vi "Terminal-ModbusEthernet-ReadInputRegisters.vi"(5 "write operation timeout (ms)":i32=5000 caption="写操作超时（毫秒）", 7 "read operation timeout (ms)":i32=5000 caption="读操作超时（毫秒）", 8 "error in":errorcluster, 9 "number of input registers":u16 caption="输入寄存器数量", 10 "starting address":u16 caption="起始地址", 11 "unit ID":u8 caption="单元ID") -> (0 "error out":errorcluster, 3 "register values":u16[](array[numeric]) caption="寄存器值")   [LabVIEW 2014]
uses:
  <vilib>/Modbus/subvis/Modbus API/Modbus API.lvclass/Modbus API.ctl
  <vilib>/Modbus/subvis/Transmission Data Unit (ADU)/Transmission Data Unit/Transmission Data Unit.lvclass/Transmission Data Unit.ctl
  <vilib>/Modbus/master/Data Access/Unit ID/Set Unit ID Property.vi
  <vilib>/Modbus/subvis/Transmission Data Unit (ADU)/Transmission Data Unit/Data Access/Unit ID/Write Unit ID.vi
  <vilib>/Modbus/subvis/Modbus API/Read Transmission Data Unit.vi
  <vilib>/Modbus/subvis/Modbus API/Write Transmission Data Unit.vi
  Configuration-Global.vi
  <vilib>/Modbus/master/Create Master Instance (TCP).vi
  <vilib>/Modbus/subvis/Transmission Data Unit (ADU)/Transmission Data Unit/Transmission Data Unit.lvclass
  <vilib>/Modbus/master/Modbus Master.lvclass
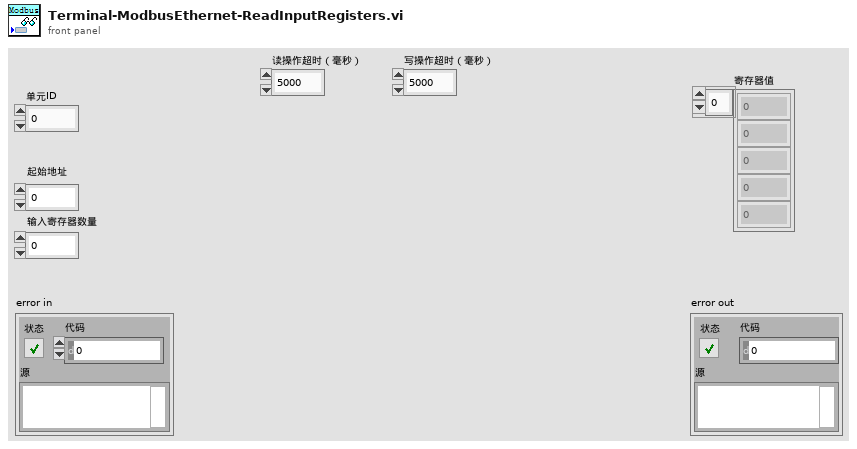
[diagram p1: front panel]
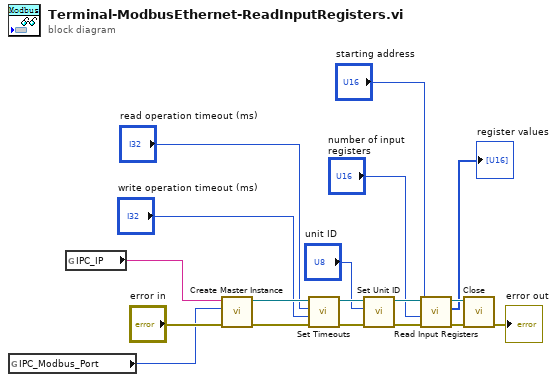
[diagram p0: block diagram]
diagram:
  n1 = global read "Configuration-Global.vi" "IPC_Modbus_Port"() -> (w4:i32)
  n2 = global read "Configuration-Global.vi" "IPC_IP"() -> (w5:string)
  n3 = call-poly <vilib>:"Create Master Instance.vi"("error in (no error)"="error in", "port (502)"=w4, "address"=w5) -> ("error out"=w16:errorcluster, "TCP master instance"=w15:refnum<class "Modbus Master.lvclass">)  [unwired: 7 in]
  n4 = call <vilib>:"Set Timeouts.vi"("error in (no error)"=w16, "write operation timeout (ms)"="write operation timeout (ms)", "read operation timeout (ms)"="read operation timeout (ms)", "Modbus master in"=w15) -> ("error out"=w7:errorcluster, "Modbus master out"=w17:refnum<class "Modbus Master.lvclass">)  [unwired: 6 in]
  n5 = call <vilib>:"Set Unit ID.vi"("error in (no error)"=w7, "unit ID"="unit ID", "Modbus master in"=w17) -> ("error out"=w9:errorcluster, "Modbus master out"=w8:refnum<class "Modbus Master.lvclass">)  [unwired: 7 in]
  n6 = call-dynamic "Read Input Registers.vi"("error in (no error)"=w9, "number of input registers"="number of input registers", "starting address"="starting address", "Modbus master in"=w8) -> ("error out"=w11:errorcluster, "register values"=→"register values":u16[], "Modbus master out"=w12:refnum<class "Modbus Master.lvclass">)  [unwired: 5 in]
  n7 = call-dynamic "Close.vi"("error in (no error)"=w11, "Modbus master in"=w12) -> ("error out"=→"error out":errorcluster)  [unwired: 9 in]
